vi "hardwarecalinit.vi"   [LabVIEW 2009]
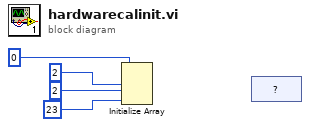
[diagram p0: block diagram]
diagram:
  n1 = Initialize Array(u8 0, 2 ("dimension size"), 2 ("dimension size"), 23 ("dimension size")) -> ()  [unwired: 1 out]
  n2 = shared-variable "?"() -> ()  [unwired: 1 in, 2 out]
